vi "MCAWindowold.vi"(8 "Ch1 Livetime":dbl, 9 "Ch0 Livetime":dbl, 10 "Histogram Data":u32[][](array[numeric]), 11 "Window":i32[](array[numeric])) -> (0 "Ch1 Rate":dbl=19.909942866187833, 1 "Ch1 Counts":u32=199, 2 "Ch0 Rate":dbl=19.81108025794395, 3 "Ch0 Counts":u32=198)   [LabVIEW 2011]
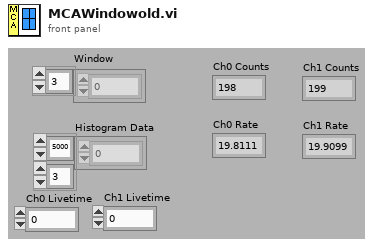
[diagram p1: front panel]
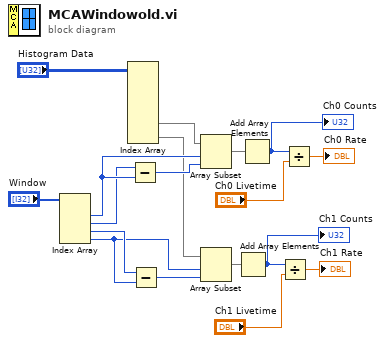
[diagram p0: block diagram]
diagram:
  n1 = Index Array(array="Window") -> (element #1=w6:i32, element #2=w5:i32, element #3=w4:i32, element #4=w3:i32)  [unwired: 4 in]
  n2 = Index Array(array="Histogram Data") -> (element #3=w1:u32[], element #4=w2:u32[])  [unwired: 8 in, 2 out]
  n3 = Subtract(x=w5, y=w6) -> (x-y=w9:i32)
  n4 = Subtract(x=w4, y=w3) -> (x-y=w14:i32)
  n5 = Array Subset(array=w1, index=w6, length=w9) -> (w10:u32[])
  n6 = Array Subset(array=w2, index=w3, length=w14) -> (w15:u32[])
  n7 = Add Array Elements(numeric array=w15) -> (sum=w16:u32)
  "Ch1 Counts" <- w16
  n8 = Add Array Elements(numeric array=w10) -> (sum=w11:u32)
  "Ch0 Counts" <- w11
  n9 = Divide(x=w16, y="Ch1 Livetime") -> (x/y=→"Ch1 Rate":dbl)
  n10 = Divide(x=w11, y="Ch0 Livetime") -> (x/y=→"Ch0 Rate":dbl)
